vi "Write Terminal.vi"(8 "Error In":errorcluster, 10 "Terminal":T1, 11 "Channel In":refnum<class "Channel.lvclass">) -> (0 "Error Out":errorcluster, 3 "Channel Out":refnum<class "Channel.lvclass">)   [LabVIEW 2018, in "Toolkit.lvlib" / "Channel.lvclass"]
uses:
  Channel.lvclass
  Typedefs/Terminals.ctl
  Channel.lvclass/Channel.ctl
  Session/Session.lvclass/Session.ctl
  SSH/SSH.lvclass/SSH.ctl
  Session/Session.lvclass
  Toolkit.lvlib
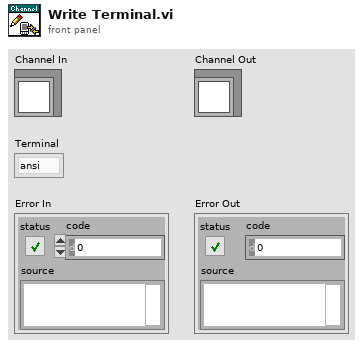
[diagram p1: front panel]
types:
  T1 = typedef "Toolkit.lvlib/Channel.lvclass/Terminals.ctl" = enum16{"ansi", "dump", "linux", "rxvt", "screen", "sun", "vt100", "vt102", "vt220", "vt52", "xterm"}
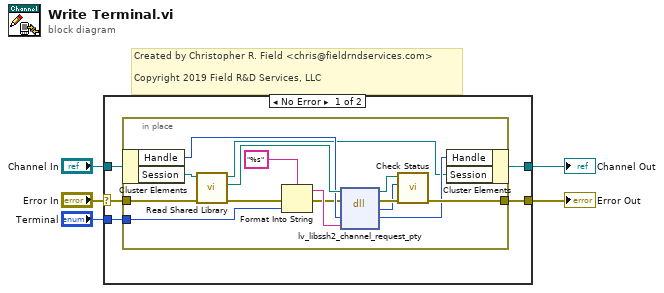
[diagram p0: block diagram]
diagram:
  # "Created by Christopher R. Field <chris@fieldrndservices.com>\n\nCopyright 2019 Field R&D Services, LLC"
  n1 = case shown="No Error" "Error In" {
    selector: "Error In" -> [w8 w27]
    tunnel: [w7 w27] -> w4
    tunnel: "Channel In" -> [w10 w26]
    tunnel: [w9 w26] -> w2
    tunnel: "Terminal" -> [w6 _]
    frame No Error {
      n2 = in-place {
        in-place-border: w8 -> [w23]
        in-place-border: [w19] -> w7
        in-place-border: w6 -> [w14]
        n3 = in-place-cluster #1(w10) -> ("Handle"=w18:u64, "Session"=w25:refnum<class "Session.lvclass">)
        n4 = call "Read Shared Library.vi"("Error In"=w23, "Session In"=w25) -> ("Erorr Out"=w15:errorcluster, "libssh2lv Shared Library"=w24:path, "Session Out"=w16:refnum<class "Session.lvclass">)  [unwired: 7 in]
        n5 = Format Into String(format string="%s", error in=w15, w14) -> (resulting string=w12:string, error out=w11:errorcluster)  [unwired: 1 in]
        n6 = dll-call lib="libssh2lv.*" fn="lv_libssh2_channel_request_pty"(path in=w24, error in=w11, "handle"=w18, "terminal"=w12) -> (path out=w21:path, error out=w22:errorcluster, "status"=w20:i32, "handle"=w17:u64)  [unwired: 2 in]
        n7 = call "Check Status.vi"("Error In"=w22, "Status"=w20, "lv-libssh2 Shared Library In"=w21) -> ("Error Out"=w19:errorcluster)  [unwired: 7 in, 1 out]
        n8 = in-place-cluster #1("Handle"=w17, "Session"=w16) -> (w9:refnum<class "Channel.lvclass">)
      }
    }
    frame Error {
    }
  }
  "Error Out" <- w4
  "Channel Out" <- w2
